vi "FTW-Example-TransferClient.vi"() -> ()   [LabVIEW 2014]
panel:
  in  "Local Destination Filepath":path=path "%UserDesktop%/test.txt"
  out "Current Rate":dbl format="%_3pbytes/sec"
  out "Iterations":i32
  out "AbsoluteURI":string
  out "Est. Time Remaining":dbl format="%.1f sec"
  out "Cancelled?":bool
  out "Local Destination":path
  out "error out":errorcluster
  in  "Remote URI":string="ftp://ftp.ni.com/evaluation/labview/MotionAssistant250.exe"
  out "Total Size (bytes)":dbl format="%_4p"
  out "Error Message":string
  out "Error?":bool
  out "Percent Done":dbl(slide) scale=0.0..100.0
  in  "Cancel Download":bool
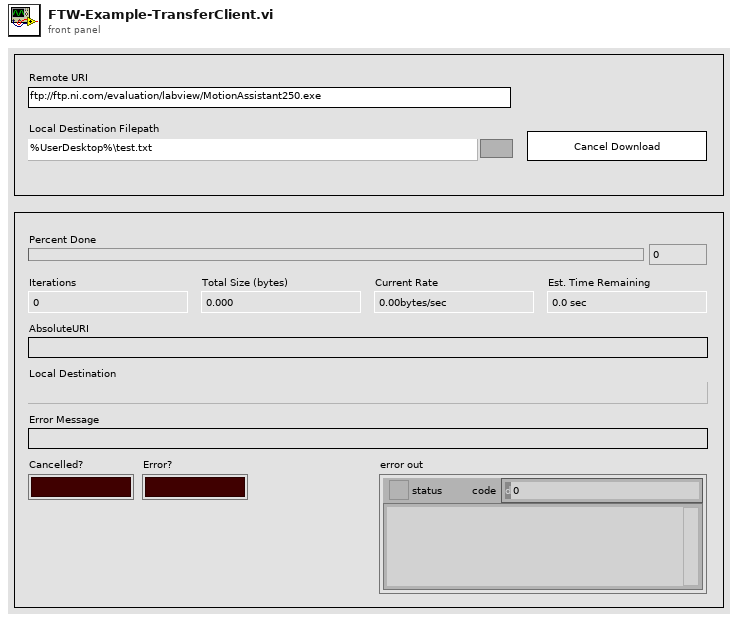
[diagram p1: front panel]
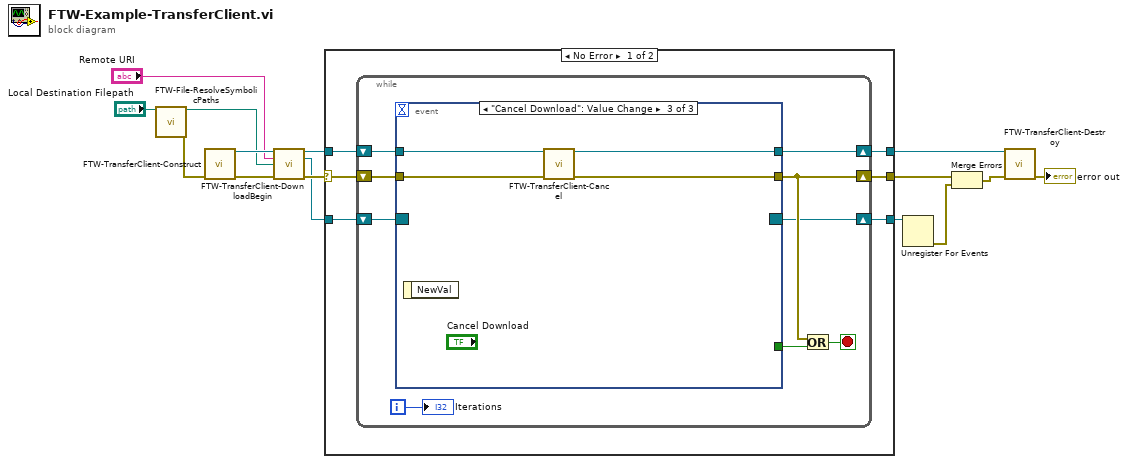
[diagram p0: block diagram]
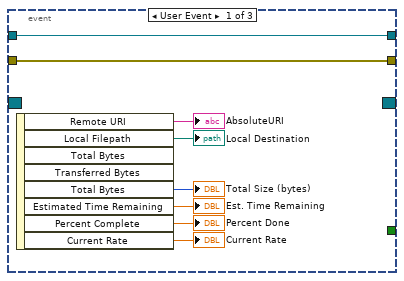
[diagram p2: hidden frame]
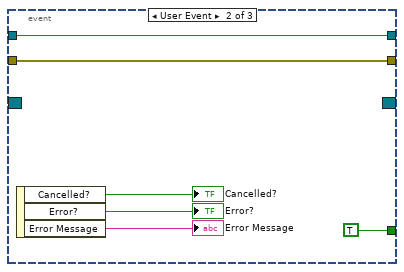
[diagram p3: hidden frame]
diagram:
  n1 = call "FTW-File-ResolveSymbolicPaths.vi"("Unresolved Path"="Local Destination Filepath") -> ("Resolved Path"=w2:path, "error out"=w1:errorcluster)  [unwired: 13 in]
  n2 = call "FTW-TransferClient-Construct.vi"("error in"=w1) -> ("Transfer Client"=w9:refnum<k24>, "error out"=w7:errorcluster)  [unwired: 13 in]
  n3 = call "FTW-TransferClient-DownloadBegin.vi"("Transfer Client"=w9, "Remote URI"="Remote URI", "Local Filepath"=w2, "error in"=w7) -> ("Transfer Client out"=w8:refnum<k24>, "Download Events"=w5:refnum<event-registration>, "error out"=w6:errorcluster)  [unwired: 9 in]
  n4 = case shown="No Error" w6 {
    selector: w6 -> [w18 w50]
    tunnel: w8 -> [w21 w51]
    tunnel: [w16 w49] -> w15
    tunnel: [w20 w51] -> w14
    tunnel: [w19 w50] -> w12
    tunnel: w5 -> [w17 w49]
    frame No Error {
      n5 = while {
        shift-right: [w28] -> w20
        shift-left: w21 -> [w30]
        shift-right: [w26] -> w19
        shift-left: w18 -> [w29]
        shift-right: [w22] -> w16
        shift-left: w17 -> [w23]
        i -> [w24]
        stop <- w25 stop-if-true
        n6 = event shown="[2] \"Cancel Download\": Value Change" {
          selector: w23 -> [_ _ _]
          dyn-events: [_ _ _] -> w22
          timeout: _ -> [_ _ _]
          tunnel: w30 -> [w37 w42 w48]
          tunnel: [w36 w40 w46] -> w26
          tunnel: w29 -> [w36 w40 w47]
          tunnel: [w37 w42 w45] -> w28
          tunnel: [_ TRUE _] -> w27
          event User Event {
            n7 = event-data() -> ("Remote URI"=→"AbsoluteURI":string, "Local Filepath"=→"Local Destination":path, "Total Bytes"=→"Total Size (bytes)":i64, "Estimated Time Remaining"=→"Est. Time Remaining":dbl, "Percent Complete"=→"Percent Done":dbl, "Current Rate"=→"Current Rate":dbl)  [unwired: 1 in, 2 out]
          }
          event User Event {
            n8 = event-data() -> ("Cancelled?"=→"Cancelled?":bool, "Error?"=→"Error?":bool, "Error Message"=→"Error Message":string)  [unwired: 1 in]
          }
          event "Cancel Download": Value Change {
            n9 = event-data() -> ()  [unwired: 1 in, 1 out]
            n10 = call "FTW-TransferClient-Cancel.vi"("Transfer Client"=w48, "error in"=w47) -> ("Transfer Client out"=w45:refnum<k24>, "error out"=w46:errorcluster)  [unwired: 12 in]
          }
        }
        n11 = Or(x=w26, y=w27) -> (x .or. y?=w25:bool)
        "Iterations" <- w24
      }
    }
    frame Error {
    }
  }
  n12 = Unregister For Events(event registration refnum=w15) -> (error out=w11:errorcluster)  [unwired: 1 in]
  n13 = Merge Errors(w12, w11) -> (w10:errorcluster)
  n14 = call "FTW-TransferClient-Destroy.vi"("Transfer Client"=w14, "error in"=w10) -> ("error out"=→"error out":errorcluster)  [unwired: 13 in]
